vi "setI32.vi"(8 "error in (no error)":errorcluster, 9 "Data":i32, 10 "Index":i32, 11 "FixedFrameBuilder in":refnum<class "FixedFrameBuilder.lvclass">) -> (0 "error out":errorcluster, 3 "FixedFrameBuilder out":refnum<class "FixedFrameBuilder.lvclass">)   [LabVIEW 2015, in "RTModbus.lvlib" / "FixedFrameBuilder.lvclass"]
uses:
  FixedFrameBuilder.lvclass
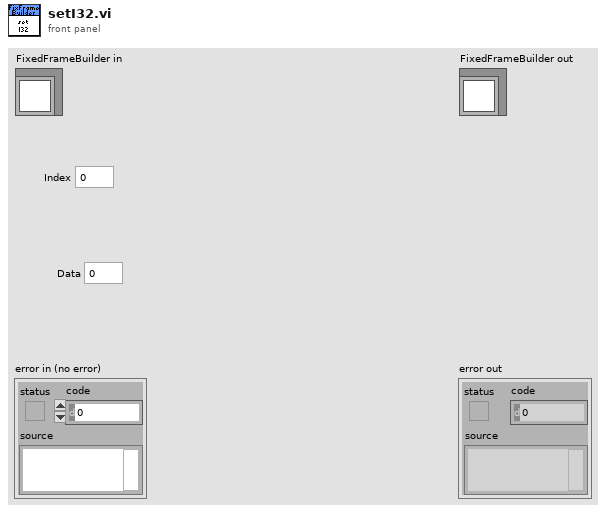
[diagram p1: front panel]
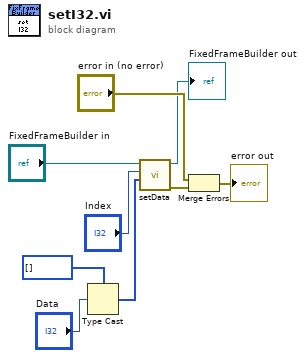
[diagram p0: block diagram]
diagram:
  n1 = Type Cast(type=u8[] [], x="Data") -> (*(type *) &x=w6:u8[])
  n2 = call "setData.vi"("Data"=w6, "Index"="Index", "FixedFrameBuilder in"="FixedFrameBuilder in") -> ("error out"=w5:errorcluster, "FixedFrameBuilder out"=→"FixedFrameBuilder out":refnum<class "FixedFrameBuilder.lvclass">)  [unwired: 7 in]
  n3 = Merge Errors("error in (no error)", w5) -> (→"error out":errorcluster)
